vi "MQTT_TCP_Open_Connection.vi"(6 "local port (0)":u16, 8 "error in (no error)":errorcluster, 9 "timeout ms (20000)":i32=20000, 10 "remote port or service name":u16=1883, 11 "address":string="broker.mqttdashboard.com") -> (0 "error out":errorcluster, 3 "connection ID":refnum<k5>)   [LabVIEW 2019]
panel:
  # "this is just a wrapper for the TCP Connect function\nadd or replace functionality as desired"
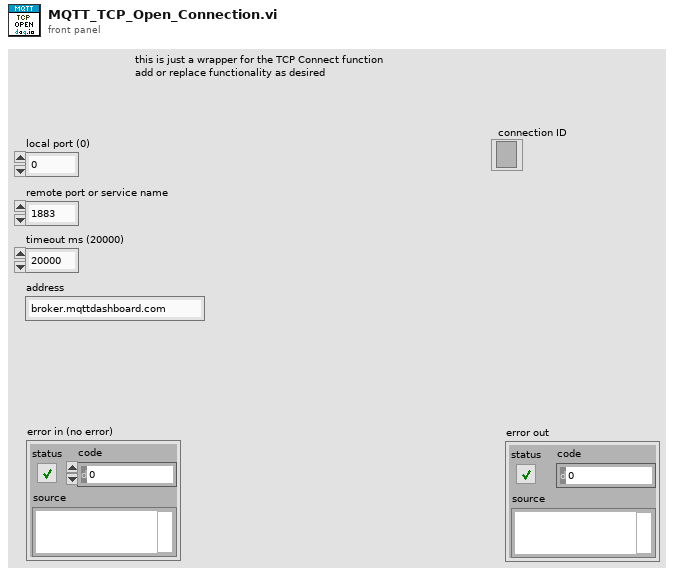
[diagram p1: front panel]
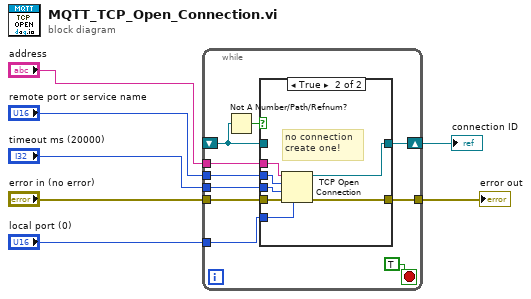
[diagram p0: block diagram]
diagram:
  n1 = while {
    tunnel: "local port (0)" -> [w17]
    tunnel: "error in (no error)" -> [w16]
    tunnel: "timeout ms (20000)" -> [w15]
    tunnel: "remote port or service name" -> [w10]
    tunnel: "address" -> [w14]
    tunnel: [w13] -> w2
    shift-right: [w12] -> w1
    shift-left: _ -> [w8]
    stop <- TRUE stop-if-true
    n2 = Not A Number/Path/Refnum?(number/path/refnum=w8) -> (NaN/Path/Refnum?=w9:bool)
    n3 = case shown="True" w9 {
      tunnel: w17 -> [_ w26]
      tunnel: w16 -> [w18 w25]
      tunnel: w15 -> [_ w24]
      tunnel: w10 -> [_ w23]
      tunnel: w14 -> [_ w22]
      tunnel: [w18 w21] -> w13
      tunnel: [w19 w20] -> w12
      tunnel: w8 -> [w19 _]
      frame False {
        # "retrieve last \nconnection ID"
      }
      frame True {
        # "no connection\ncreate one!"
        n4 = TCP Open Connection(address=w22, remote port or service name=w23, timeout ms (60000)=w24, local port=w26, error in (no error)=w25) -> (connection ID=w20:refnum<k5>, error out=w21:errorcluster)
      }
    }
  }
  "error out" <- w2
  "connection ID" <- w1
